vi "DataAcquireParameters.vi"(0 "Start position":dbl, 5 "Target position":dbl, 7 "Velocity":dbl) -> (3 "Rate":dbl, 4 "Start Position":dbl, 6 "Target Position":dbl, 8 "Range":dbl, 10 "Velocity":dbl, 13 "Movement direction":string, 14 "Number of Samples":i32, 15 "Time":dbl)   [LabVIEW 2013]
uses:
  Global.vi
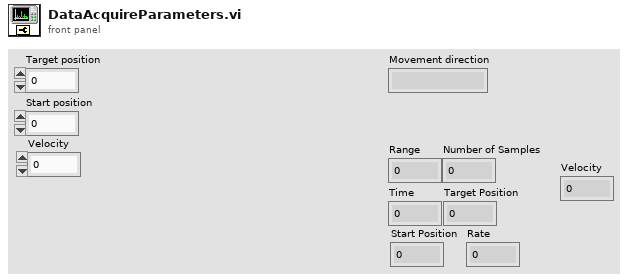
[diagram p1: front panel]
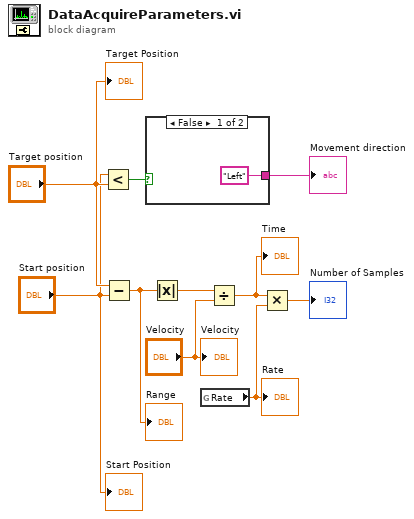
[diagram p0: block diagram]
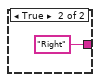
[diagram p2: hidden frame]
diagram:
  n1 = Less?(x="Start position", y="Target position") -> (x < y?=w7:bool)
  n2 = Subtract(x="Target position", y="Start position") -> (x-y=w2:dbl)
  "Range" <- w2
  n3 = case shown="False" w7 {
    tunnel: ["Left" "Right"] -> w6
    frame False {
    }
    frame True {
    }
  }
  "Movement direction" <- w6
  n4 = Absolute Value(x=w2) -> (abs(x)=w1:dbl)
  n5 = global read "Global.vi" "Rate"() -> (w9:dbl)
  "Rate" <- w9
  n6 = Divide(x=w1, y="Velocity") -> (x/y=w10:dbl)
  "Time" <- w10
  n7 = Multiply(x=w10, y=w9) -> (x*y=→"Number of Samples":dbl)
  "Target Position" <- "Target position"
  "Start Position" <- "Start position"
  "Velocity" <- "Velocity"
